vi "Rec Get Value From Field.vi"(6 "error in (no error)":errorcluster, 8 "column index":variant, 9 "recordset reference":T1) -> (0 "error out":errorcluster, 2 "value":variant, 3 "recordset reference out":T1)   [LabVIEW 2020, in "NI_Database_API.lvlib"]
doc: "Gets the value located at the <B>column index</B> of the current record in the recordset identified by the recordset reference. The <B>column index</B> can either be the zero-indexed position of the column in the recordset or the name of the column."
uses:
  <vilib>/addons/database/NI_Database_API.lvlib
  <vilib>/addons/database/Recordset.llb/Rec ObjectReference.ctl
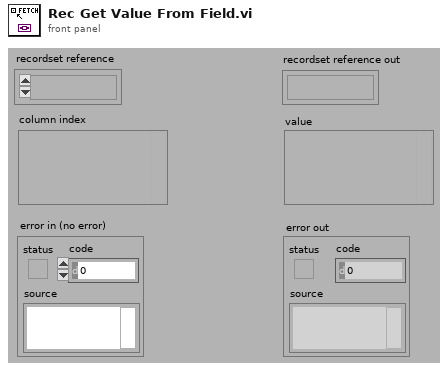
[diagram p1: front panel]
types:
  T1 = typedef "NI_Database_API.lvlib/Rec ObjectReference.ctl" = refnum<k1>
  T2 = typedef "NI_Database_API.lvlib/Rec DataMembers.ctl" = cluster{"ADODB._Recordset":refnum<k7>, "Connection":T3}
  T3 = typedef "NI_Database_API.lvlib/Conn ObjectReference.ctl" = refnum<k1>
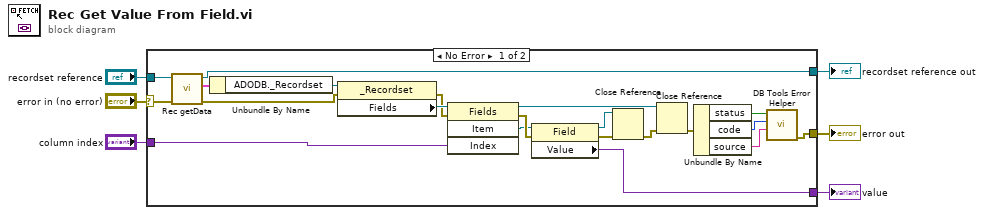
[diagram p0: block diagram]
diagram:
  n1 = case shown="No Error" "error in (no error)" {
    selector: "error in (no error)" -> [w7 w29]
    tunnel: [w27 _] -> w6
    tunnel: [w22 w28] -> w5
    tunnel: "recordset reference" -> [w19 w28]
    tunnel: "column index" -> [w18 _]
    tunnel: [w8 w29] -> w2
    frame No Error {
      n2 = call <vilib>:"Rec getData.vi"("error in (no error)"=w7, "recordset reference"=w19) -> ("error out"=w23:errorcluster, "data"=w21:T2, "recordset reference out"=w22:T1)  [unwired: 3 out]
      n3 = Unbundle By Name(w21) -> ("ADODB._Recordset"=w13:refnum<k7>)
      n4 = property class="_Recordset"(reference=w13, error in=w23) -> (error out=w20:errorcluster, "Fields"=w24:refnum<k7>)  [unwired: 1 out]
      n5 = invoke class="Fields" method="Item"(reference=w24, error in=w20, "Index"=w18) -> (reference out=w15:refnum<k7>, error out=w17:errorcluster, "Item"=w14:refnum<k7>)  [unwired: 1 in, 1 out]
      n6 = property class="Field"(reference=w14, error in=w17) -> (reference out=w26:refnum<k7>, error out=w25:errorcluster, "Value"=w27:variant)
      n7 = Close Reference(reference=w26, error in (no error)=w25) -> (error out=w16:errorcluster)
      n8 = Close Reference(reference=w15, error in (no error)=w16) -> (error out=w9:errorcluster)
      n9 = Unbundle By Name(w9) -> ("status"=w11:bool, "code"=w10:i32, "source"=w12:string)
      n10 = call <vilib>:"DB Tools Error Helper.vi"("source"=w12, "code"=w10, "status"=w11) -> ("error out"=w8:errorcluster)  [unwired: 1 in, 7 out]
    }
    frame Error {
    }
  }
  "value" <- w6
  "error out" <- w2
  "recordset reference out" <- w5
